vi "加密解密字符串（映射表）.vi"(7 "映射表":u8[](array[numeric])=[149, 131, 111, 218, 161, 223, 167, 96, 220, 194, 178, 70, 162, 32, 128, 158, 14, 135, 242, 151, 35, 236, 79, 213, 168, 202, 105, 69, 143, 172, 51, 73, 67, 20, 248, 235, 48, 41, 212, 85, 241, 90, 123, 91, 110, 29, 118, 254, 68, 246, 100, 87, 219, 157, 7, 17, 66, 94, 120, 55, 75, 240, 145, 109, 54, 141, 82, 1, 127, 146, 3, 22, 193, 81, 227, 65, 150, 6, 132, 189, 229, 83, 214, 148, 12, 226, 113, 25, 74, 176, 58, 101, 185, 27, 98, 50, 197, 204, 224, 233, 152, 228, 63, 243, 18, 4, 190, 57, 155, 53, 62, 163, 23, 122, 124, 217, 46, 255, 16, 187, 112, 102, 169, 133, 200, 59, 191, 13, 31, 33, 139, 231, 92, 137, 232, 103, 210, 24, 177, 249, 78, 142, 159, 134, 247, 116, 199, 165, 34, 245, 222, 47, 144, 56, 130, 195, 196, 170, 225, 38, 198, 126, 15, 10, 76, 2, 108, 11, 121, 64, 239, 203, 21, 154, 37, 39, 117, 206, 140, 138, 174, 188, 72, 180, 156, 173, 99, 252, 5, 129, 36, 147, 221, 251, 80, 211, 19, 215, 237, 77, 183, 208, 9, 238, 43, 253, 42, 52, 28, 45, 104, 8, 160, 184, 95, 61, 97, 40, 106, 44, 71, 93, 153, 205, 164, 201, 30, 86, 136, 26, 244, 179, 171, 175, 107, 250, 234, 186, 119, 216, 192, 0, 166, 182, 230, 49, 60, 207, 125, 114, 88, 209, 89, 84, 181, 115], 8 "error in (no error)":errorcluster caption="错误输入（无错误）", 9 "模式":enum16{"加密", "解密"}(ring), 11 "输入字符串":string) -> (0 "error out":errorcluster caption="错误输出", 3 "输出字符串":string)   [LabVIEW 2012]
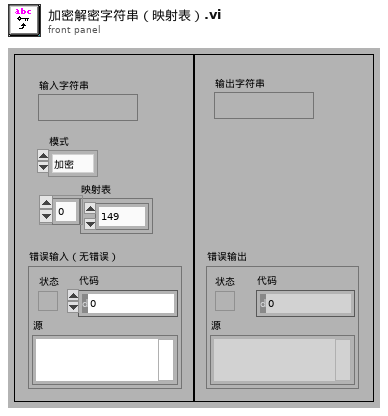
[diagram p1: front panel]
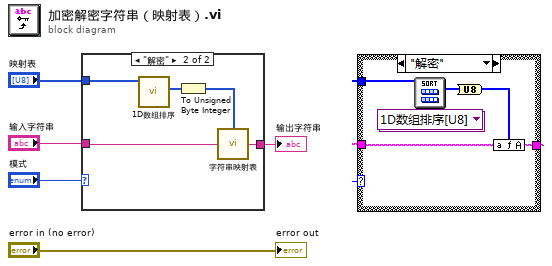
[diagram p0: block diagram]
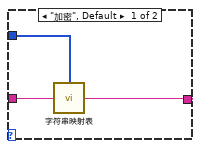
[diagram p2: hidden frame]
diagram:
  n1 = case shown="\"解密\"" "模式" {
    tunnel: "映射表" -> [w8 w13]
    tunnel: "输入字符串" -> [w7 w10]
    tunnel: [w6 w9] -> w4
    frame "加密", Default {
      n2 = call "字符串映射表.vi"("输入字符串"=w7, "映射表"=w8) -> ("输出字符串"=w6:string)
    }
    frame "解密" {
      n3 = call-poly "1D数组排序.vi"("输入数组"=w13) -> ("排序后索引"=w12:i32[])  [unwired: 8 in, 2 out]
      n4 = To Unsigned Byte Integer(number=w12) -> (unsigned 8bit integer=w11:u8[])
      n5 = call "字符串映射表.vi"("输入字符串"=w10, "映射表"=w11) -> ("输出字符串"=w9:string)
    }
  }
  "输出字符串" <- w4
  "error out" <- "error in (no error)"
